vi "GetOutputWireBranch.vi"(6 "error in":errorcluster, 9 "Tunnel in":refnum<class "FlatSequenceOuterTunnel.lvclass">) -> (0 "error out":errorcluster, 3 "Tunnel out":refnum<class "FlatSequenceOuterTunnel.lvclass">, 4 "branches":string, 5 "branched":bool)   [LabVIEW 2014, in "Raspberry Pi Compatible Compiler for LabVIEW.lvlib" / "FlatSequenceOuterTunnel.lvclass"]
uses:
  FlatSequenceOuterTunnel.lvclass
  FlatSequenceOuterTunnel.lvclass/FlatSequenceOuterTunnel.ctl
  Terminal/Terminal.lvclass
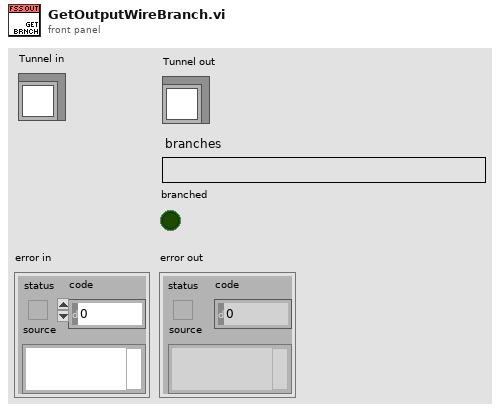
[diagram p1: front panel]
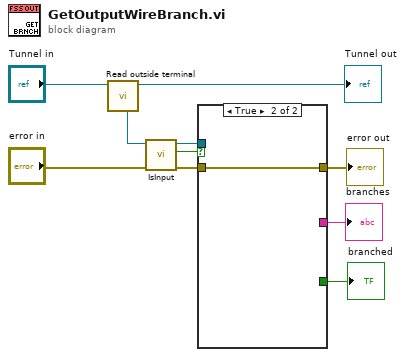
[diagram p0: block diagram]
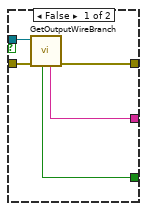
[diagram p2: hidden frame]
diagram:
  n1 = call "Read outside terminal.vi"("FlatSequenceInnerTunnel in"="Tunnel in") -> ("FlatSequenceInnerTunnel out"=→"Tunnel out":refnum<class "FlatSequenceOuterTunnel.lvclass">, "outside terminal"=w3:refnum<class "Terminal.lvclass">)  [unwired: 7 in]
  n2 = call-dynamic "IsInput.vi"("error in"="error in", "Terminal in"=w3) -> ("error out"=w5:errorcluster, "input"=w1:bool, "Terminal out"=w4:refnum<class "Terminal.lvclass">)  [unwired: 5 in]
  n3 = case shown="True" w1 {
    tunnel: [w15 _] -> w8
    tunnel: [w14 _] -> w7
    tunnel: [w13 w16] -> w6
    tunnel: w5 -> [w12 w16]
    tunnel: w4 -> [w11 _]
    frame False {
      n4 = call-dynamic "GetOutputWireBranch.vi"("error in"=w12, "Terminal in"=w11) -> ("error out"=w13:errorcluster, "branches"=w15:string, "branched"=w14:bool)  [unwired: 4 in, 1 out]
    }
    frame True {
    }
  }
  "error out" <- w6
  "branches" <- w8
  "branched" <- w7
